vi "写入COM.vi"(8 "error in (no error)":errorcluster caption="错误输入（无错误）", 10 "COM":refnum<visa-resource-name>, 11 "通讯输入":refnum<class "通讯.lvclass">) -> (0 "error out":errorcluster caption="错误输出", 3 "通讯输出":refnum<class "通讯.lvclass">)   [LabVIEW 2015, in "通讯.lvlib" / "通讯.lvclass"]
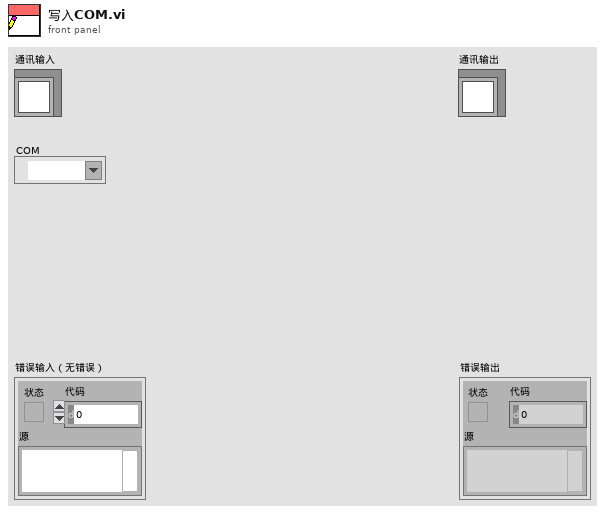
[diagram p1: front panel]
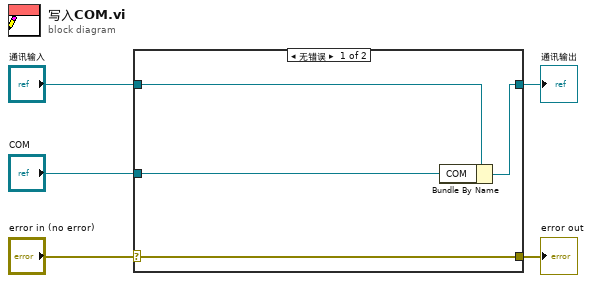
[diagram p0: block diagram]
diagram:
  n1 = case shown="无错误" "error in (no error)" {
    selector: "error in (no error)" -> [w9 w10]
    tunnel: [w9 w10] -> w4
    tunnel: [w7 w11] -> w2
    tunnel: "通讯输入" -> [w8 w11]
    tunnel: "COM" -> [w6 _]
    frame No Error {
      n2 = Bundle By Name(cluster=w8, "COM"=w6) -> (w7:refnum<class "通讯.lvclass">)
    }
    frame Error {
    }
  }
  "error out" <- w4
  "通讯输出" <- w2
